vi "UI.vi"(8 "error":errorcluster, 11 "2-axis":refnum<class "Syncronus 2-Axis Stage.lvclass">) -> (0 "error out":errorcluster)   [LabVIEW 2022 SP3, in "JKI UI.lvlib"]
uses:
  JKI UI.lvlib
  Syncronus 2-Axis Stage/Syncronus 2-Axis Stage.lvclass
panel:
  out "XY Position Graph":cluster{"X":dbl, "Y":dbl}[](graph)
  in  "Clear Error":bool
  in  "Set X-Speed":u16
  in  "Set Y-Speed":u16
  in  "Set X-Acceleration":u16
  in  "Set Y-Acceleration":u16
  out "X-Speed":dbl
  out "Y-Speed":dbl
  out "X-Current Speed":dbl
  out "Y-Current Speed":dbl
  out "X-Acceleration":dbl
  out "Y-Acceleration":dbl
  out "Y-Homed":bool
  out "X-Homed":bool
  out "X-Moving":bool
  out "Y-Moving":bool
  out "Y-Position":dbl
  out "X-Position":dbl
  out "Stage Error":errorcluster
  in  "Abort Motion":bool
  in  "Home Stage":bool
  in  "Move Stage":bool
  in  "Y-Destination":dbl
  in  "X-Destination":dbl
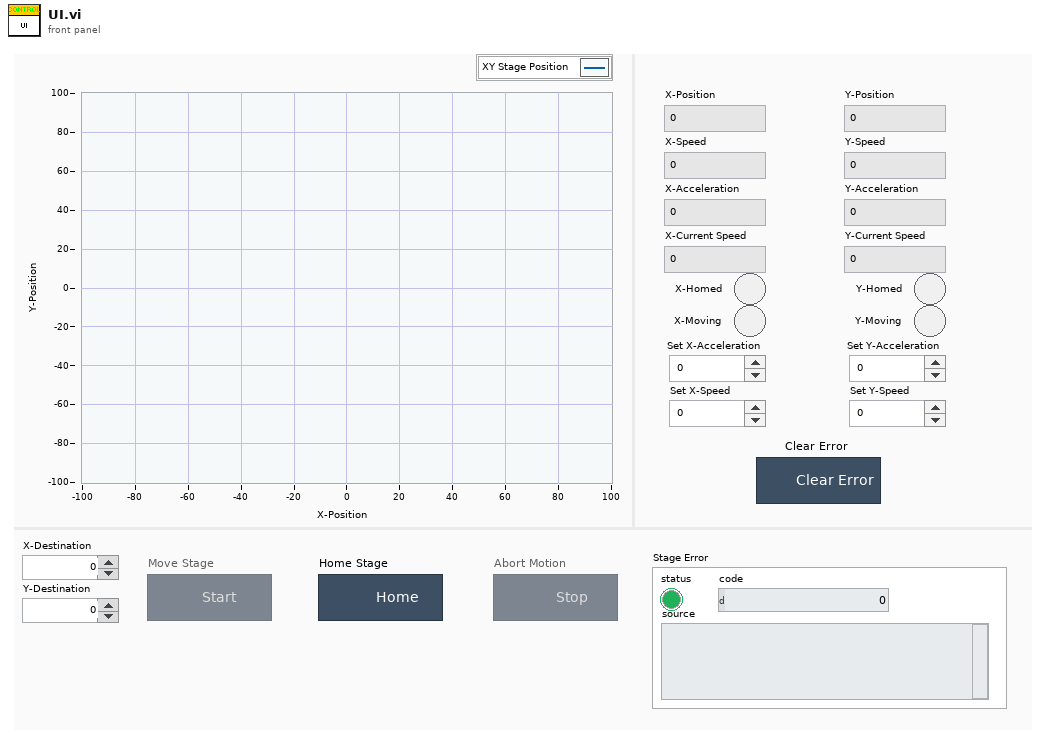
[diagram p1: front panel]
types:
  T1 = enum32{"Invalid", "Standard", "Closed", "Hidden", "Minimized", "Maximized"}
  T2 = enum32{"invalid app kind", "Development System", "Run Time System", "Student Edition", "Embedded LabVIEW", "Evaluation", "Custom"}
  T3 = enum8{"Enabled", "Disabled", "Disabled and Grayed Out"}
  T4 = cluster{"Core":cluster{"Current VI Reference":refnum<vi>, "Close Panel on Exit?":bool}, "2-axis":refnum<class "Syncronus 2-Axis Stage.lvclass">}
  T5 = cluster{"Current VI Reference":refnum<vi>, "Close Panel on Exit?":bool}
  T6 = cluster{"Current Position X":dbl, "Current Position Y":dbl}[]
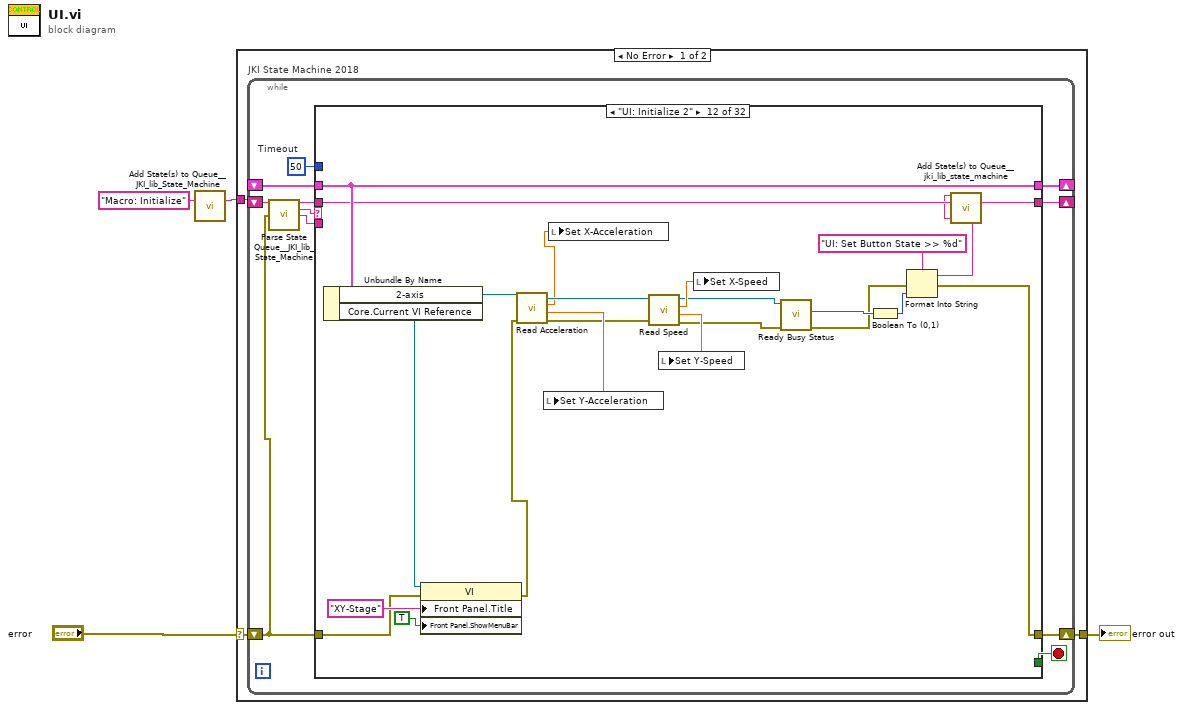
[diagram p0: block diagram]
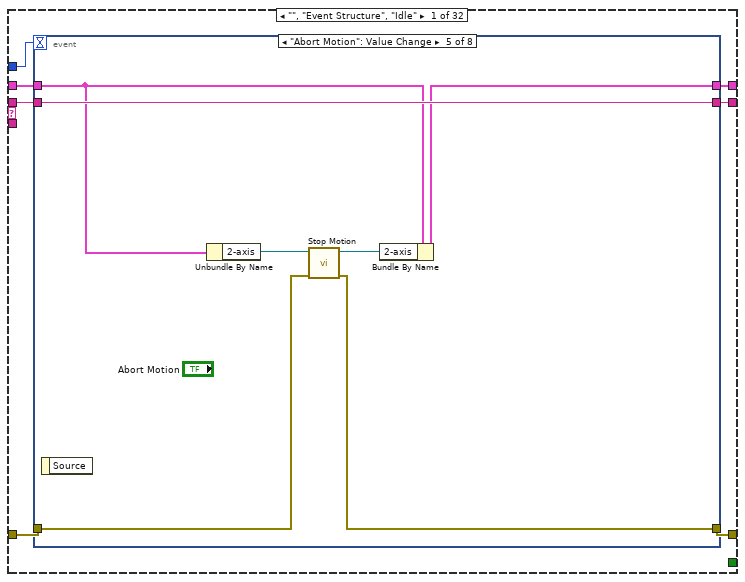
[diagram p2: hidden frame]
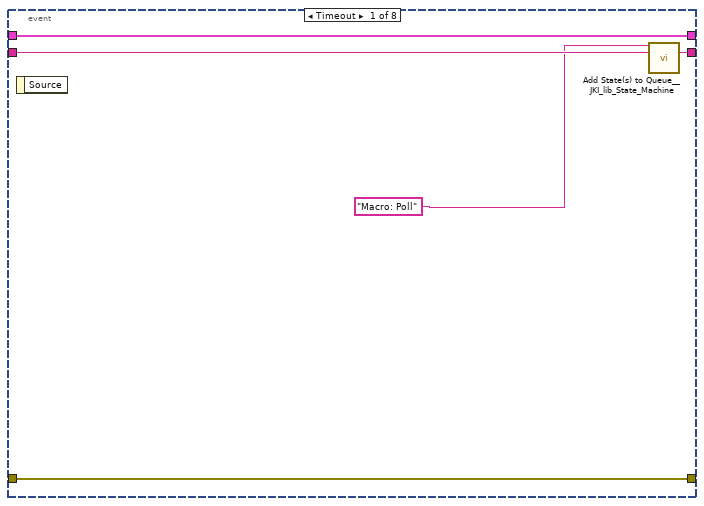
[diagram p3: hidden frame]
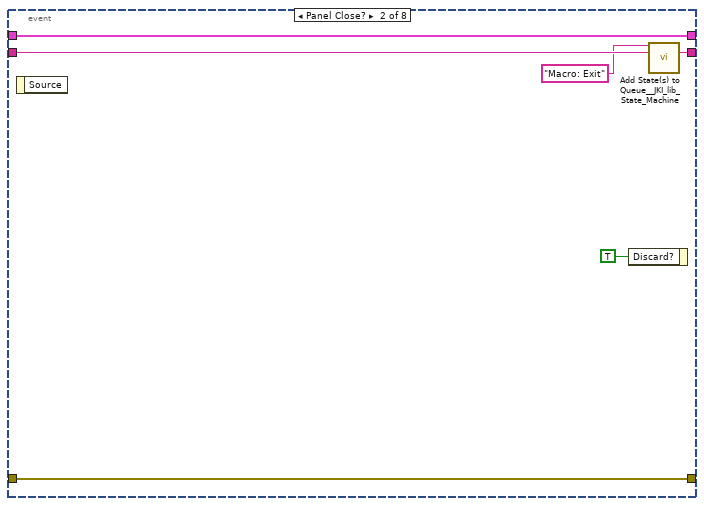
[diagram p4: hidden frame]
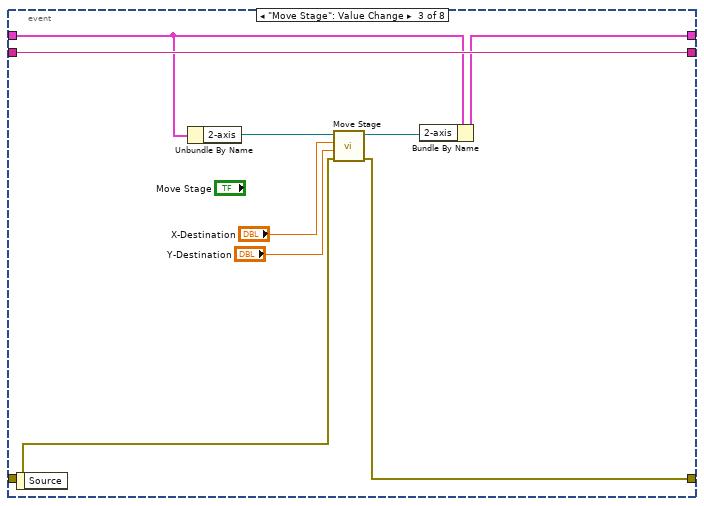
[diagram p5: hidden frame]
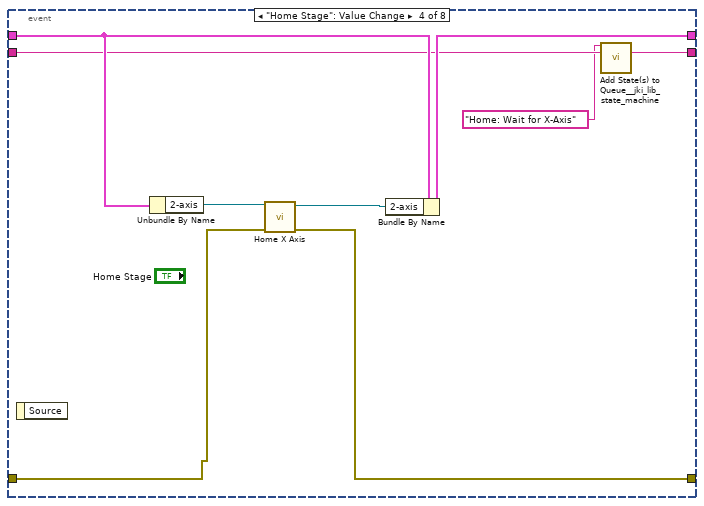
[diagram p6: hidden frame]
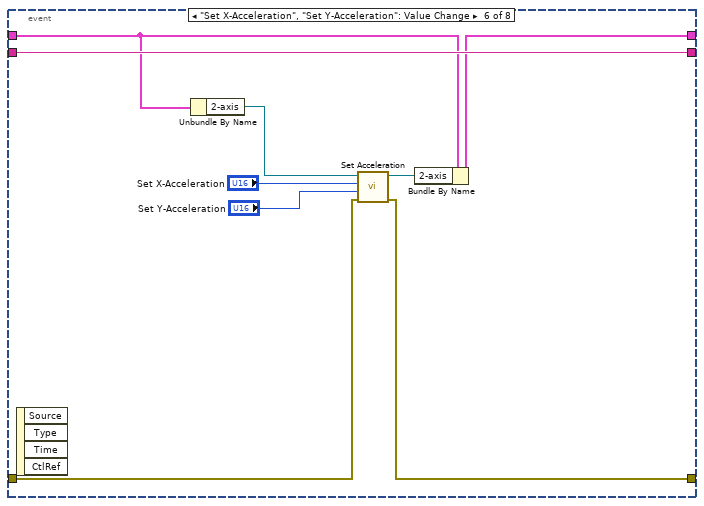
[diagram p7: hidden frame]
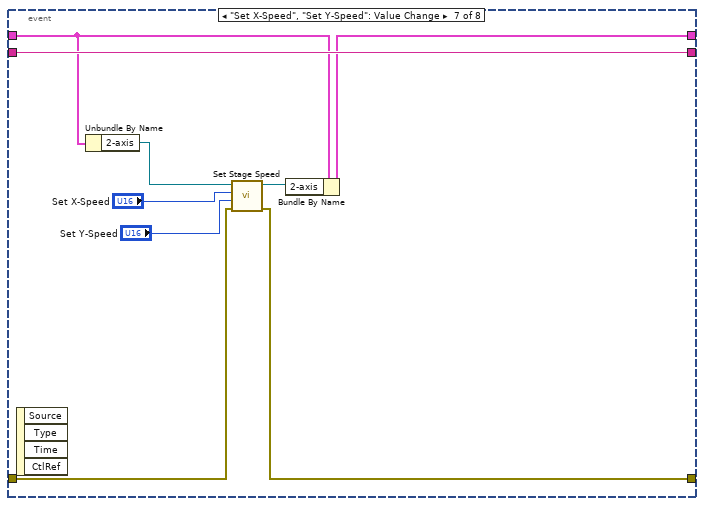
[diagram p8: hidden frame]
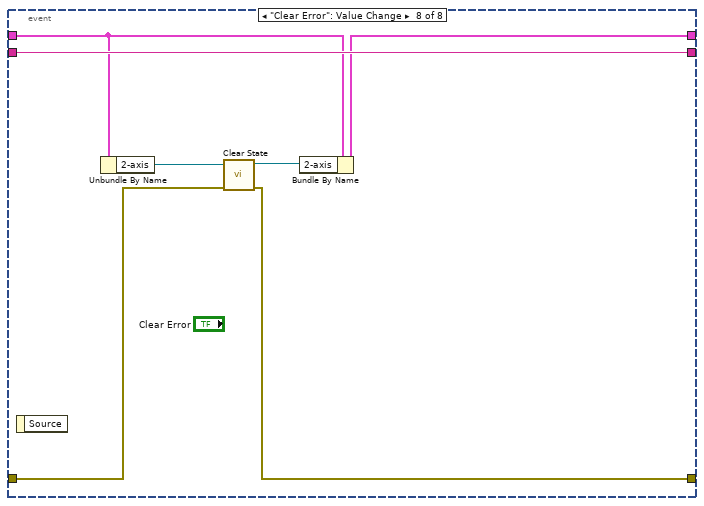
[diagram p9: hidden frame]
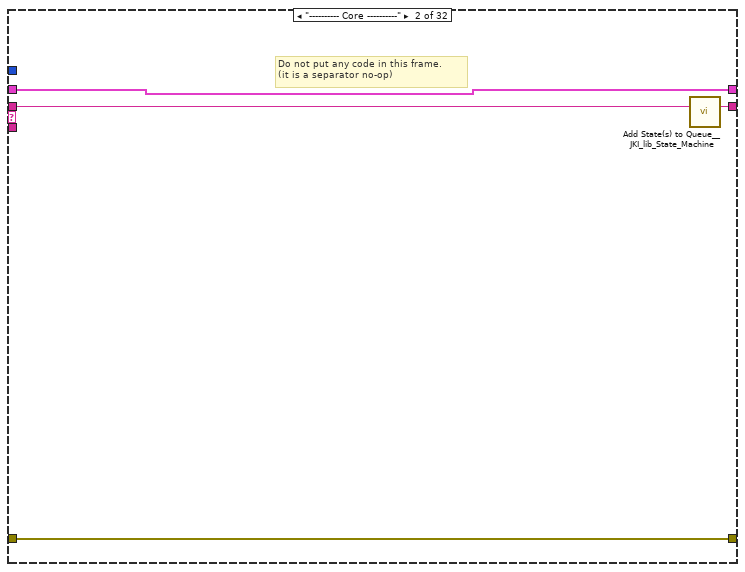
[diagram p10: hidden frame]
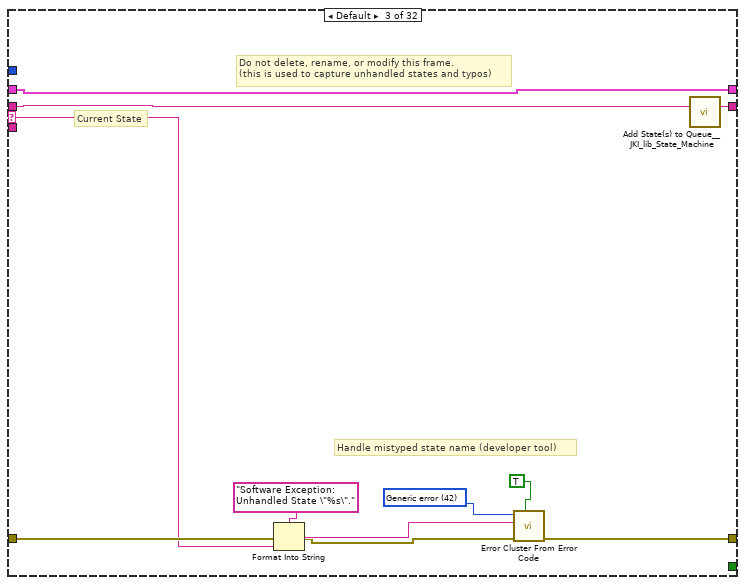
[diagram p11: hidden frame]
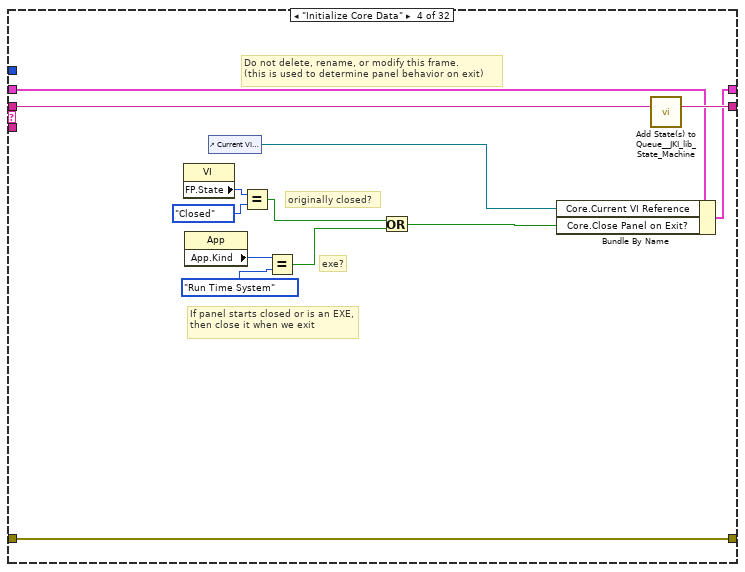
[diagram p12: hidden frame]
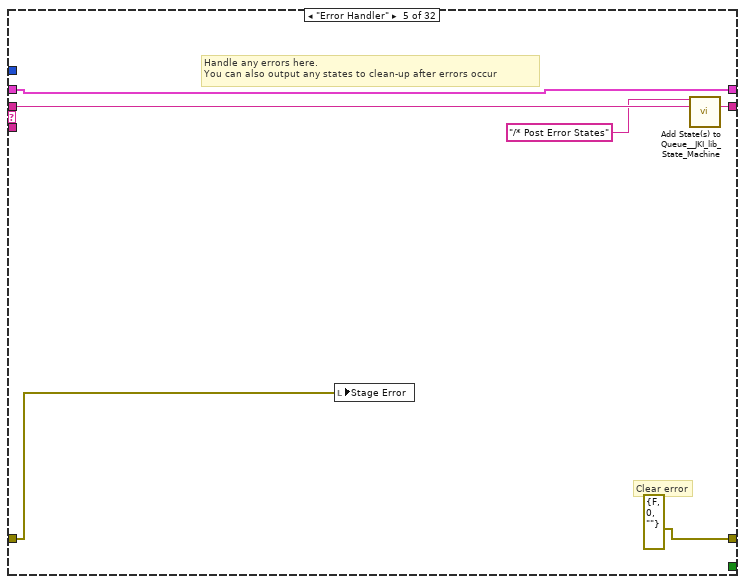
[diagram p13: hidden frame]
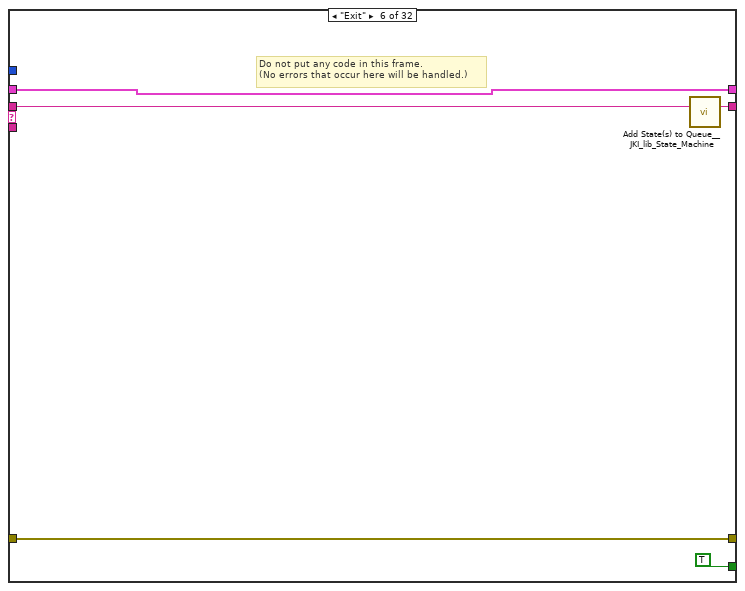
[diagram p14: hidden frame]
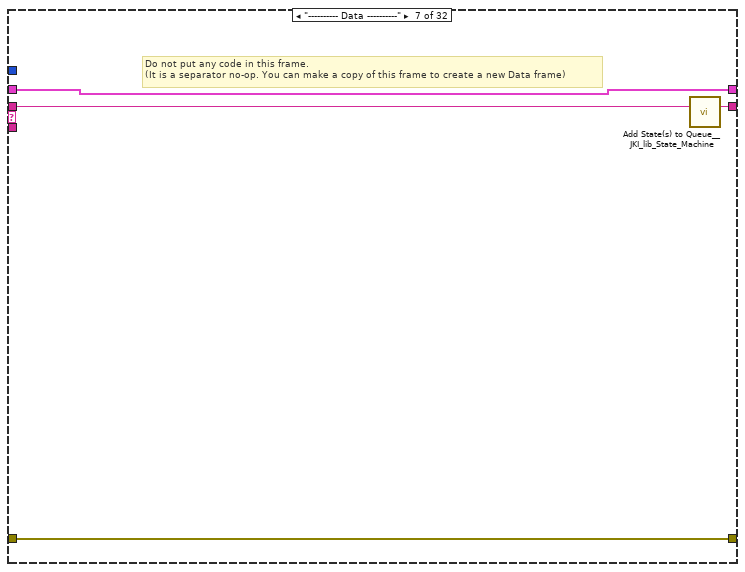
[diagram p15: hidden frame]
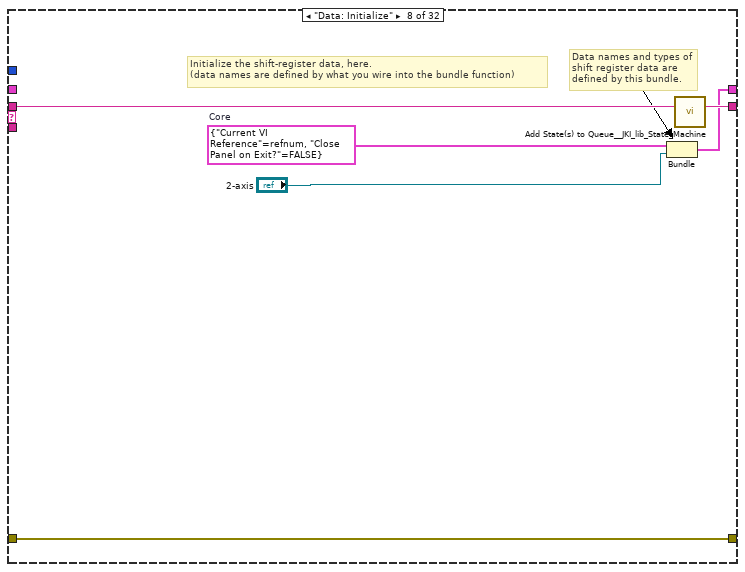
[diagram p16: hidden frame]
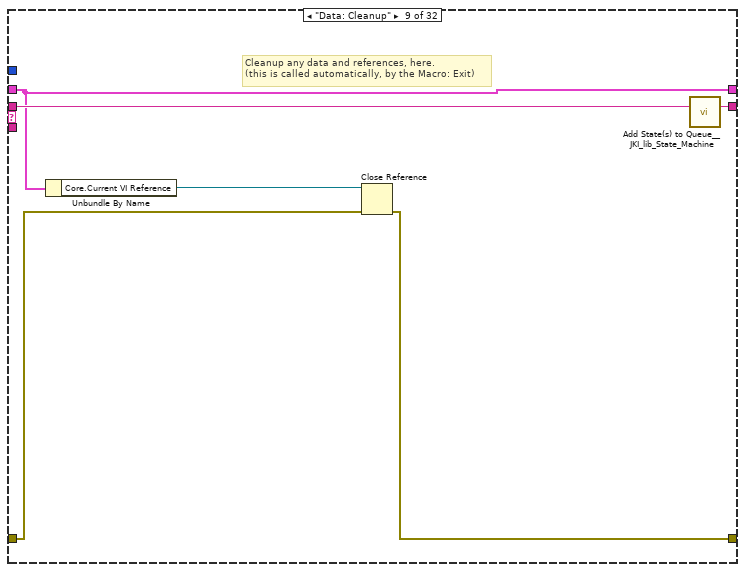
[diagram p17: hidden frame]
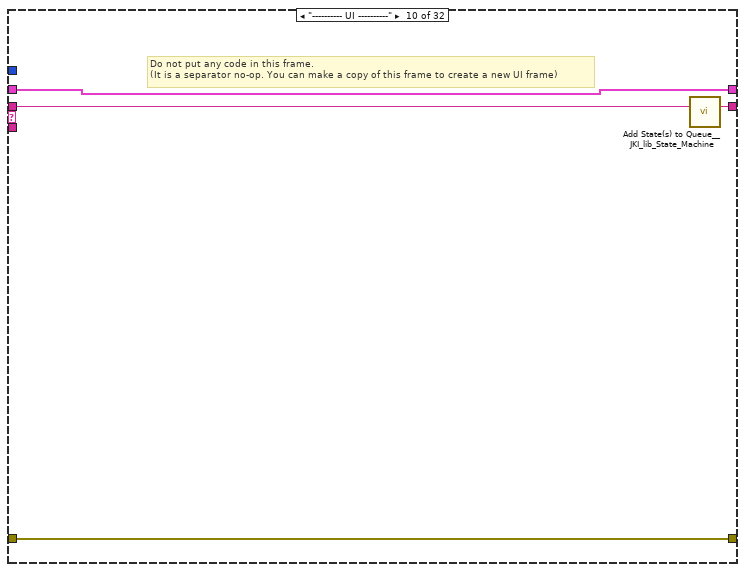
[diagram p18: hidden frame]
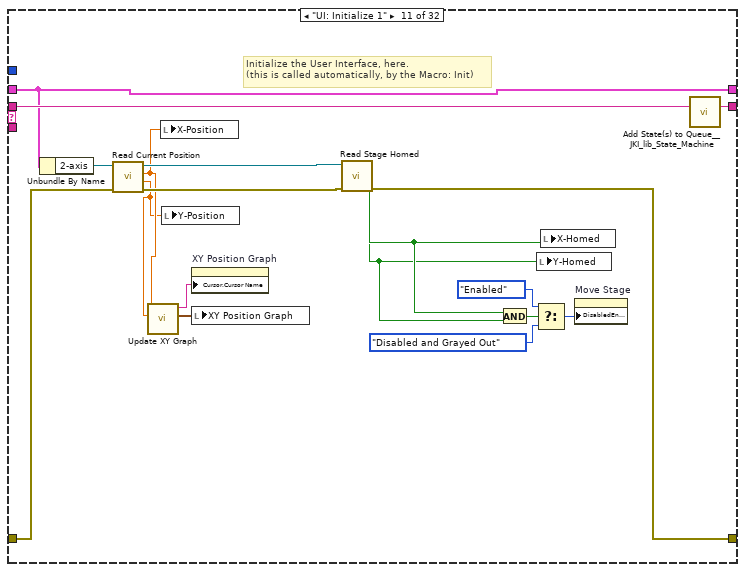
[diagram p19: hidden frame]
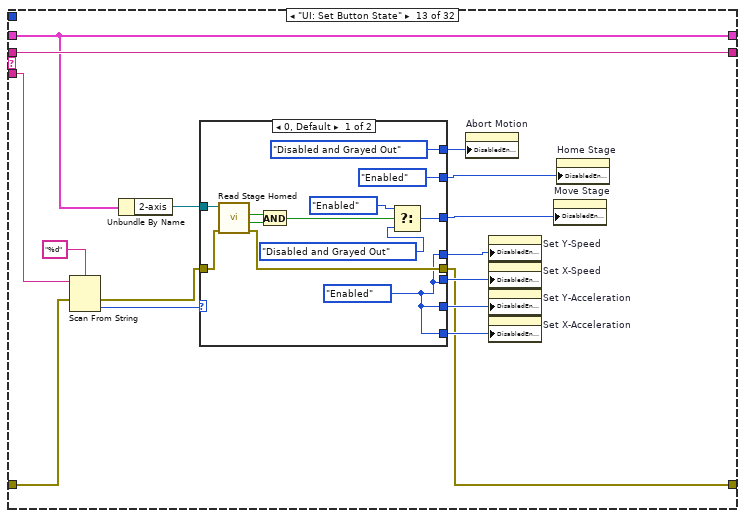
[diagram p20: hidden frame]
diagram:
  n1 = call <vilib>:"Add State(s) to Queue__JKI_lib_State_Machine.vi"("State(s) in (\"\")"="Macro: Initialize") -> ("States Out"=w1:string)  [unwired: 14 in]
  n2 = case shown="No Error" "error" {
    selector: "error" -> [w7 _]
    tunnel: [w6 _] -> w3
    tunnel: w1 -> [w5 _]
    frame No Error {
      n3 = while "JKI State Machine 2018" {
        shift-right: [w11] -> _
        shift-left: _ -> [w10]
        shift-right: [w14] -> w6
        shift-left: w7 -> [w8]
        shift-right: [w13] -> _
        shift-left: w5 -> [w15]
        stop <- w12 stop-if-true
        w9 = 50  # Timeout
        n4 = call <vilib>:"Parse State Queue__JKI_lib_State_Machine.vi"("State Queue"=w15, "Error In (no error)"=w8) -> ("Remaining States"=w17:string, "Current State"=w18:string, "Arguments"=w16:string)  [unwired: 11 in]
        n5 = case shown="\"UI: Initialize 2\"" w18 {
          selector: w18 -> [_ _ w91 _ _ _ _ _ _ _ _ _ _ _ _ _ _ _ _ _ _ _ _ _ _ _ _ _ _ _ _ _]
          tunnel: w17 -> [w25 w90 w95 w114 w120 w125 w129 w135 w141 w145 w163 w184 w202 w223 w234 w303 w308 w318 w321 w326 w338 w347 w356 w365 w374 w380 w395 w403 w406 w413 w433 w442]
          tunnel: w16 -> [_ _ _ _ _ _ _ _ _ _ _ _ w192 w218 w228 _ _ _ _ _ _ _ _ _ _ _ _ _ _ _ _ _]
          tunnel: w10 -> [w23 w87 w93 w107 w117 w123 w126 _ w136 w142 w161 w186 w194 w221 w230 w300 w305 w315 w323 w325 w335 w346 w355 w364 w373 w384 w394 w402 w405 w423 w440 w449]
          tunnel: [w22 w88 w97 w111 errorcluster {"status"=FALSE, "code"=0, "source"=""} ("error out") w122 w127 w132 w137 w143 w151 w165 w189 w219 w231 w301 w306 w316 w319 w324 w329 w341 w350 w359 w368 w377 w391 w398 w404 w409 w425 w446] -> w14
          tunnel: w8 -> [w21 w88 w96 w111 w115 w122 w127 w132 w138 w143 w158 w170 w188 w220 w232 w301 w306 w316 w319 w324 w331 w342 w351 w360 w369 w378 w392 w399 w404 w411 w427 w447]
          tunnel: [w24 w89 w94 w113 w119 w124 w128 w134 w140 w144 w162 w185 w202 w222 w233 w302 w307 w317 w322 w326 w338 w347 w356 w365 w374 w381 w395 w403 w406 w414 w434 w443] -> w13
          tunnel: [_ _ _ _ _ TRUE _ _ _ _ _ _ _ _ _ _ _ _ _ _ _ _ _ _ _ _ _ _ _ _ _ _] -> w12
          tunnel: [w20 w87 w93 w112 w117 w123 w126 w133 w136 w142 w161 w186 w194 w221 w230 w300 w305 w315 w323 w325 w328 w340 w349 w358 w367 w376 w388 w397 w405 w408 w429 w445] -> w11
          tunnel: w9 -> [w19 _ _ _ _ _ _ _ _ _ _ _ _ _ _ _ _ _ _ _ _ _ _ _ _ _ _ _ _ _ _ _]
          frame "", "Event Structure", "Idle" {
            n6 = event shown="[4] \"Abort Motion\": Value Change" {
              selector: _ -> [_ _ _ _ _ _ _ _]
              dyn-events: _ -> [_ _ _ _ _ _ _ _]
              timeout: w19 -> [_ _ _ _ _ _ _ _]
              tunnel: w25 -> [w30 w36 w45 w47 w61 w70 w79 w86]
              tunnel: [w29 w35 w45 w48 w61 w70 w79 w86] -> w24
              tunnel: w23 -> [w27 w33 w44 w54 w60 w69 w78 w85]
              tunnel: [w28 w34 w40 w49 w59 w65 w76 w83] -> w22
              tunnel: w21 -> [w28 w34 w41 w50 w58 w66 w77 w84]
              tunnel: [w27 w33 w38 w53 w56 w63 w72 w81] -> w20
              event Timeout {
                n7 = event-data() -> ()  [unwired: 1 in, 1 out]
                n8 = call <vilib>:"Add State(s) to Queue__JKI_lib_State_Machine.vi"("State(s) in Front (\"\")"="Macro: Poll", "State(s) in (\"\")"=w30) -> ("States Out"=w29:string)  [unwired: 13 in]
              }
              event Panel Close? {
                n9 = event-data() -> ()  [unwired: 1 in, 1 out]
                n10 = event-data("Discard?"=TRUE) -> ()  [unwired: 1 in, 1 out]
                n11 = call <vilib>:"Add State(s) to Queue__JKI_lib_State_Machine.vi"("State(s) in Front (\"\")"="Macro: Exit", "State(s) in (\"\")"=w36) -> ("States Out"=w35:string)  [unwired: 13 in]
              }
              event "Move Stage": Value Change {
                n12 = event-data() -> ()  [unwired: 1 in, 1 out]
                n13 = Unbundle By Name(w44) -> ("2-axis"=w39:refnum<class "Syncronus 2-Axis Stage.lvclass">)
                n14 = call-dynamic "Move Stage.vi"("error in (no error)"=w41, "Y Axis"="Y-Destination", "X Axis"="X-Destination", "2-Axis Stage in"=w39) -> ("error out"=w40:errorcluster, "2-Axis Stage out"=w37:refnum<class "Syncronus 2-Axis Stage.lvclass">)  [unwired: 6 in]
                n15 = Bundle By Name(cluster=w44, "2-axis"=w37) -> (w38:T4)
              }
              event "Home Stage": Value Change {
                n16 = event-data() -> ()  [unwired: 1 in, 1 out]
                n17 = Unbundle By Name(w54) -> ("2-axis"=w52:refnum<class "Syncronus 2-Axis Stage.lvclass">)
                n18 = call-dynamic "Home X Axis.vi"("error in (no error)"=w50, "Synchronous Home in"=w52) -> ("error out"=w49:errorcluster, "Synchronous Home out"=w51:refnum<class "Syncronus 2-Axis Stage.lvclass">)  [unwired: 8 in]
                n19 = Bundle By Name(cluster=w54, "2-axis"=w51) -> (w53:T4)
                n20 = call <vilib>:"Add State(s) to Queue__jki_lib_state_machine.vi"("State(s) in Front (\"\")"="Home: Wait for X-Axis" ("State(s) in Front (\"\")"), "State(s) in (\"\")"=w47) -> ("States Out"=w48:string)  [unwired: 13 in]
              }
              event "Abort Motion": Value Change {
                n21 = event-data() -> ()  [unwired: 1 in, 1 out]
                n22 = Unbundle By Name(w60) -> ("2-axis"=w57:refnum<class "Syncronus 2-Axis Stage.lvclass">)
                n23 = call-dynamic "Stop Motion.vi"("error in (no error)"=w58, "2-Axis Stage in"=w57) -> ("error out"=w59:errorcluster, "2-Axis Stage out"=w55:refnum<class "Syncronus 2-Axis Stage.lvclass">)  [unwired: 8 in]
                n24 = Bundle By Name(cluster=w60, "2-axis"=w55) -> (w56:T4)
              }
              event "Set X-Acceleration", "Set Y-Acceleration": Value Change {
                n25 = event-data() -> ()  [unwired: 1 in, 4 out]
                n26 = Unbundle By Name(w69) -> ("2-axis"=w64:refnum<class "Syncronus 2-Axis Stage.lvclass">)
                n27 = call-dynamic "Set Acceleration.vi"("error in (no error)"=w66, "Y Axis"="Set Y-Acceleration", "X Axis"="Set X-Acceleration", "2-Axis Stage in"=w64) -> ("error out"=w65:errorcluster, "2-Axis Stage out"=w62:refnum<class "Syncronus 2-Axis Stage.lvclass">)  [unwired: 6 in]
                n28 = Bundle By Name(cluster=w69, "2-axis"=w62) -> (w63:T4)
              }
              event "Set X-Speed", "Set Y-Speed": Value Change {
                n29 = event-data() -> ()  [unwired: 1 in, 4 out]
                n30 = Unbundle By Name(w78) -> ("2-axis"=w73:refnum<class "Syncronus 2-Axis Stage.lvclass">)
                n31 = call-dynamic "Set Stage Speed.vi"("error in (no error)"=w77, "Y Axis"="Set Y-Speed", "X Axis"="Set X-Speed", "2-Axis Stage in"=w73) -> ("error out"=w76:errorcluster, "2-Axis Stage out"=w71:refnum<class "Syncronus 2-Axis Stage.lvclass">)  [unwired: 6 in]
                n32 = Bundle By Name(cluster=w78, "2-axis"=w71) -> (w72:T4)
              }
              event "Clear Error": Value Change {
                n33 = event-data() -> ()  [unwired: 1 in, 1 out]
                n34 = Unbundle By Name(w85) -> ("2-axis"=w82:refnum<class "Syncronus 2-Axis Stage.lvclass">)
                n35 = call-dynamic "Clear State.vi"("error in (no error)"=w84, "2-Axis Stage Status in"=w82) -> ("error out"=w83:errorcluster, "2-Axis Stage Status out"=w80:refnum<class "Syncronus 2-Axis Stage.lvclass">)  [unwired: 8 in]
                n36 = Bundle By Name(cluster=w85, "2-axis"=w80) -> (w81:T4)
              }
            }
          }
          frame "---------- Core ----------" {
            # "Do not put any code in this frame.\n(it is a separator no-op)"
            n37 = call <vilib>:"Add State(s) to Queue__JKI_lib_State_Machine.vi"("State(s) in (\"\")"=w90) -> ("States Out"=w89:string)  [unwired: 14 in]
          }
          frame Default {
            w100 = 42 items=["No error", "Argument error", "Memory is full", "Out of zone", "End of file", "File already open", "Generic file I/O error", "File not found", "File permission error", "Disk is full", "Duplicate path", "Too many files open", "System feature not enabled", "Resource file not found", "Cannot add resource", "Resource not found", "Image not found", "Image memory error", "Pen does not exist", "Config type invalid", "Config token not found", "Config parse error", "Config memory error", "Bad external code format", "Bad external code offset", "External code not present", "Null window", "Destroy window error", "Null menu", "Print aborted", "Bad print record", "Print driver error", "Windows error during printing", "Memory error during printing", "Print dialog error", "Generic print error", "Invalid device refnum", "Device not found", "Device parameter error", "Device unit error", "Cannot open device", "Device call aborted", "Generic error", "Cancelled by user", "Object ID too low", "Object ID too high", "Object not in heap", "Unknown heap", "Unknown object (invalid DefProc)", "Unknown object (DefProc not in table)", "Message out of range", "Invalid (null) method", "Unknown message", "Manager call not supported", "Bad address", "Network operation in progress", "Network operation timed out", "Connection is busy", "Network attribute not supported", "Network error", "Address in use", "System out of memory", "Connection aborted", "Connection refused", "Not connected", "Already connected", "Connection closed", "Initialization error (interapplication manager)", "Bad occurrence", "Wait on unbound occurrence handler", "Occurrence queue overflow", "Datalog type conflict", "Unused", "Unrecognized type (interapplication manager)", "Memory corrupt", "Failed to make temporary DLL", "Old CIN version", "Drag socket not found", "Failed to load drop-object", "Failed to register OLE object", "Failed to release OLE object", "Format specifier type mismatch", "Unknown format specifier", "Too few format specifiers", "Too many format specifiers", "Scan failed", "Newer CIN version", "Error converting to variant", "Runtime menu error", "Password tampered", "Variant attribute not found", "Incompatible variant data type", "Event data is not available", "Event Store is not present", "Occurrence is not found", "Event Queue is not created", "Event info is not available", "Refnum passed is NULL", "Error retrieving Class GUID", "Error retrieving CoClass GUID", "Error retrieving TypeLib GUID.", "Bad built application magic bytes.", "Specific driver is different from the specific driver associated with the Logical Name.", "There is no session opened to the class driver.", "Max Error", "MAX - Error with config objects", "MAX - Error loading configuration", "MAX - Group not supported"]
            # "Current State"
            # "Do not delete, rename, or modify this frame.\n(this is used to capture unhandled states and typos)"
            # "Handle mistyped state name (developer tool)"
            n38 = Format Into String(format string="Software Exception: Unhandled State \"%s\"." ("message"), error in=w96, w91) -> (resulting string=w99:string, error out=w98:errorcluster)  [unwired: 1 in]
            n39 = call <vilib>:"Error Cluster From Error Code.vi"("show call chain? (False)"=TRUE, "error in (no error)"=w98, "error message (\"\")"=w99, "error code (0)"=w100) -> ("error out"=w97:errorcluster)  [unwired: 5 in]
            n40 = call <vilib>:"Add State(s) to Queue__JKI_lib_State_Machine.vi"("State(s) in (\"\")"=w95) -> ("States Out"=w94:string)  [unwired: 14 in]
          }
          frame "Initialize Core Data" {
            # "Do not delete, rename, or modify this frame.\n(this is used to determine panel behavior on exit)"
            # "originally closed?"
            # "exe?"
            # "If panel starts closed or is an EXE, then close it when we exit"
            n41 = property class="VI"() -> ("FP.State"=w104:T1)  [unwired: 2 in, 2 out]
            n42 = property class="App"() -> ("App.Kind"=w110:T2)  [unwired: 2 in, 2 out]
            n43 = control-ref of="Current VI Reference"() -> (w105:refnum<vi>)
            n44 = Equal?(x=w104, y=T1."Closed" ("Front Panel Window:State")) -> (x = y?=w102:bool)
            n45 = Equal?(x=w110, y=T2."Run Time System" ("Application:Kind")) -> (x = y?=w108:bool)
            n46 = Or(x=w102, y=w108) -> (x .or. y?=w106:bool)
            n47 = Bundle By Name(cluster=w107, "Core.Current VI Reference"=w105, "Core.Close Panel on Exit?"=w106) -> (w112:T4)
            n48 = call <vilib>:"Add State(s) to Queue__JKI_lib_State_Machine.vi"("State(s) in (\"\")"=w114) -> ("States Out"=w113:string)  [unwired: 14 in]
          }
          frame "Error Handler" {
            # "Handle any errors here.\nYou can also output any states to clean-up after errors occur"
            # "Clear error"
            n49 = local write "Stage Error"(w115) -> ()
            n50 = call <vilib>:"Add State(s) to Queue__JKI_lib_State_Machine.vi"("State(s) in Front (\"\")"="/* Post Error States", "State(s) in (\"\")"=w120) -> ("States Out"=w119:string)  [unwired: 13 in]
          }
          frame "Exit" {
            # "Do not put any code in this frame.\n(No errors that occur here will be handled.)"
            n51 = call <vilib>:"Add State(s) to Queue__JKI_lib_State_Machine.vi"("State(s) in (\"\")"=w125) -> ("States Out"=w124:string)  [unwired: 14 in]
          }
          frame "---------- Data ----------" {
            # "Do not put any code in this frame.\n(It is a separator no-op. You can make a copy of this frame to create a new Data frame)"
            n52 = call <vilib>:"Add State(s) to Queue__JKI_lib_State_Machine.vi"("State(s) in (\"\")"=w129) -> ("States Out"=w128:string)  [unwired: 14 in]
          }
          frame "Data: Initialize" {
            w131 = T5 {"Current VI Reference"=refnum, "Close Panel on Exit?"=FALSE}  # Core
            # "Data names and types of shift register data are defined by this bundle."
            # "Initialize the shift-register data, here.\n(data names are defined by what you wire into the bundle function)"
            n53 = Bundle("Core"=w131, "2-axis"="2-axis") -> (w133:T4)  [unwired: 1 in]
            n54 = call <vilib>:"Add State(s) to Queue__JKI_lib_State_Machine.vi"("State(s) in (\"\")"=w135) -> ("States Out"=w134:string)  [unwired: 14 in]
          }
          frame "Data: Cleanup" {
            # "Cleanup any data and references, here.\n(this is called automatically, by the Macro: Exit)"
            n55 = Unbundle By Name(w136) -> ("Core.Current VI Reference"=w139:refnum<vi>)
            n56 = Close Reference(reference=w139, error in (no error)=w138) -> (error out=w137:errorcluster)
            n57 = call <vilib>:"Add State(s) to Queue__JKI_lib_State_Machine.vi"("State(s) in (\"\")"=w141) -> ("States Out"=w140:string)  [unwired: 14 in]
          }
          frame "---------- UI ----------" {
            # "Do not put any code in this frame.\n(It is a separator no-op. You can make a copy of this frame to create a new UI frame)"
            n58 = call <vilib>:"Add State(s) to Queue__JKI_lib_State_Machine.vi"("State(s) in (\"\")"=w145) -> ("States Out"=w144:string)  [unwired: 14 in]
          }
          frame "UI: Initialize 1" {
            # "Initialize the User Interface, here.\n(this is called automatically, by the Macro: Init)"
            n59 = Unbundle By Name(w161) -> ("2-axis"=w146:refnum<class "Syncronus 2-Axis Stage.lvclass">)
            n60 = call-dynamic "Read Current Position.vi"("error in (no error)"=w158, "2-Axis Stage Status in"=w146) -> ("error out"=w159:errorcluster, "Y Position"=w149:dbl, "X Position"=w150:dbl, "2-Axis Stage Status out"=w160:refnum<class "Syncronus 2-Axis Stage.lvclass">)  [unwired: 6 in]
            n61 = call "Update XY Graph.vi"("Current Position Y"=w149, "Current Position X"=w150) -> ("Array"=w148:T6, "String"=w147:string)  [unwired: 7 in, 1 out]
            n62 = local write "X-Position"(w150) -> ()
            n63 = local write "Y-Position"(w149) -> ()
            n64 = property on="XY Position Graph" class="XYGraph (strict)"("Cursor.Cursor Name"=w147) -> ()  [unwired: 2 in, 2 out]
            n65 = local write "XY Position Graph"(w148) -> ()
            n66 = call-dynamic "Read Stage Homed.vi"("error in (no error)"=w159, "2-Axis Stage Status in"=w160) -> ("error out"=w151:errorcluster, "Y-Axis Homed Moving"=w156:bool, "X-Axis Homed"=w157:bool)  [unwired: 6 in, 1 out]
            n67 = And(x=w157, y=w156) -> (x .and. y?=w155:bool)
            n68 = Select(t=T3."Enabled" ("Disabled"), s=w155, f=T3."Disabled and Grayed Out" ("Disabled")) -> (s? t:f=w153:T3)
            n69 = local write "Y-Homed"(w156) -> ()
            n70 = local write "X-Homed"(w157) -> ()
            n71 = property on="Move Stage" class="Bool"("DisabledEnum"=w153) -> ()  [unwired: 2 in, 2 out]
            n72 = call <vilib>:"Add State(s) to Queue__JKI_lib_State_Machine.vi"("State(s) in (\"\")"=w163) -> ("States Out"=w162:string)  [unwired: 14 in]
          }
          frame "UI: Initialize 2" {
            n73 = Unbundle By Name(w186) -> ("2-axis"=w176:refnum<class "Syncronus 2-Axis Stage.lvclass">, "Core.Current VI Reference"=w179:refnum<vi>)
            n74 = property class="VI"(reference=w179, error in=w170, "Front Panel.Title"="XY-Stage" ("Front Panel Window:Title"), "Front Panel.ShowMenuBar"=TRUE ("Front Panel Window:Show Menu Bar")) -> (error out=w169:errorcluster)  [unwired: 1 out]
            n75 = call-dynamic "Read Acceleration.vi"("error in (no error)"=w169, "2-Axis Stage Status in"=w176) -> ("error out"=w168:errorcluster, "Y Acceleration"=w173:dbl, "X Acceleration"=w174:dbl, "2-Axis Stage Status out"=w175:refnum<class "Syncronus 2-Axis Stage.lvclass">)  [unwired: 6 in]
            n76 = local write "Set Y-Acceleration"(w173) -> ()
            n77 = local write "Set X-Acceleration"(w174) -> ()
            n78 = call-dynamic "Read Speed.vi"("error in (no error)"=w168, "2-Axis Stage Status in"=w175) -> ("error out"=w167:errorcluster, "Y-Axis Speed"=w171:dbl, "X-Axis Speed"=w172:dbl, "2-Axis Stage Status out"=w164:refnum<class "Syncronus 2-Axis Stage.lvclass">)  [unwired: 6 in]
            n79 = local write "Set Y-Speed"(w171) -> ()
            n80 = local write "Set X-Speed"(w172) -> ()
            n81 = call-dynamic "Ready Busy Status.vi"("error in (no error)"=w167, "2-Axis Stage Status in"=w164) -> ("error out"=w166:errorcluster, "Busy"=w181:bool)  [unwired: 7 in, 1 out]
            n82 = Boolean To (0,1)(Boolean=w181) -> (0, 1=w180:i16)
            n83 = Format Into String(format string="UI: Set Button State >> %d", error in=w166, w180) -> (resulting string=w182:string, error out=w165:errorcluster)  [unwired: 1 in]
            n84 = call <vilib>:"Add State(s) to Queue__jki_lib_state_machine.vi"("State(s) in Front (\"\")"=w182, "State(s) in (\"\")"=w184) -> ("States Out"=w185:string)  [unwired: 13 in]
          }
          frame "UI: Set Button State" {
            n85 = Scan From String(format string="%d", input string=w192, error in=w188) -> (error out=w187:errorcluster, output 1=w190:i32)  [unwired: 2 in, 2 out]
            n86 = Unbundle By Name(w194) -> ("2-axis"=w193:refnum<class "Syncronus 2-Axis Stage.lvclass">)
            n87 = case shown="0, Default" w190 {
              tunnel: [T3."Enabled" ("Disabled") w216] -> w201
              tunnel: [T3."Disabled and Grayed Out" ("Disabled") T3."Enabled" ("Disabled")] -> w200
              tunnel: [w207 w216] -> w199
              tunnel: [w206 w215] -> w189
              tunnel: [w205 w216] -> w198
              tunnel: [w205 w216] -> w197
              tunnel: [w205 w216] -> w196
              tunnel: [w205 w216] -> w195
              tunnel: w193 -> [w203 _]
              tunnel: w187 -> [w204 w215]
              frame 0, Default {
                w205 = T3."Enabled" ("Disabled")
                n88 = call-dynamic "Read Stage Homed.vi"("error in (no error)"=w204, "2-Axis Stage Status in"=w203) -> ("error out"=w206:errorcluster, "Y-Axis Homed Moving"=w211:bool, "X-Axis Homed"=w212:bool)  [unwired: 6 in, 1 out]
                n89 = And(x=w212, y=w211) -> (x .and. y?=w210:bool)
                n90 = Select(t=T3."Enabled" ("Disabled"), s=w210, f=T3."Disabled and Grayed Out" ("Disabled")) -> (s? t:f=w207:T3)
              }
              frame 1 {
                w216 = T3."Disabled and Grayed Out" ("Disabled")
              }
            }
            n91 = property on="Abort Motion" class="Bool"("DisabledEnum"=w200) -> ()  [unwired: 2 in, 2 out]
            n92 = property on="Set Y-Speed" class="DigNum (strict)"("DisabledEnum"=w198) -> ()  [unwired: 2 in, 2 out]
            n93 = property on="Set X-Speed" class="DigNum (strict)"("DisabledEnum"=w197) -> ()  [unwired: 2 in, 2 out]
            n94 = property on="Set Y-Acceleration" class="DigNum (strict)"("DisabledEnum"=w196) -> ()  [unwired: 2 in, 2 out]
            n95 = property on="Set X-Acceleration" class="DigNum (strict)"("DisabledEnum"=w195) -> ()  [unwired: 2 in, 2 out]
            n96 = property on="Move Stage" class="Bool"("DisabledEnum"=w199) -> ()  [unwired: 2 in, 2 out]
            n97 = property on="Home Stage" class="Bool"("DisabledEnum"=w201) -> ()  [unwired: 2 in, 2 out]
          }
          frame "UI: Cursor Set" {
            # "Argument"
            # "Set and Unset Cursor Busy.\n(Usage: \"UI: Cursor Set >> Busy|Idle\")"
            n98 = case shown="\"Idle\", Default" w218 {
              tunnel: w220 -> [w225 w227]
              tunnel: [w224 w226] -> w219
              frame "Idle", Default {
                n99 = call <vilib>:"Unset Busy.vi"("error in (no error)"=w225) -> ("error out"=w224:errorcluster)  [unwired: 10 in]
              }
              frame "Busy" {
                n100 = call <vilib>:"Set Busy.vi"("error in (no error)"=w227) -> ("error out"=w226:errorcluster)  [unwired: 9 in, 1 out]
              }
            }
            n101 = call <vilib>:"Add State(s) to Queue__JKI_lib_State_Machine.vi"("State(s) in (\"\")"=w223) -> ("States Out"=w222:string)  [unwired: 14 in]
          }
          frame "UI: Front Panel State" {
            # "Argument"
            # "Set Front Panel Open or Closed\n(Usage: \"UI: Front Panel State >> Open|Close\")"
            n102 = Unbundle By Name(w230) -> ("Core.Current VI Reference"=w229:refnum<vi>)
            n103 = case shown="\"Minimize\", \"Minimized\"" w228 {
              tunnel: w232 -> [w240 w255 w266 w279 w292]
              tunnel: [w242 w256 w268 w281 w294] -> w231
              tunnel: w229 -> [w241 w253 w267 w280 w293]
              frame "Open", "Standard", Default {
                w235 = T1."Standard" ("State")
                n104 = property class="VI"(reference=w241, error in=w240) -> (reference out=w238:refnum<vi>, error out=w239:errorcluster, "FP.State"=w237:T1)
                n105 = Not Equal?(x=w237, y=w235) -> (x != y?=w236:bool)
                n106 = case shown="True" w236 {
                  tunnel: [w246 w248] -> w242
                  tunnel: w239 -> [w245 w248]
                  tunnel: w238 -> [w244 _]
                  tunnel: w235 -> [w243 _]
                  frame True {
                    n107 = invoke class="VI" method="FP.Open"(reference=w244, error in=w245, "Activate"=TRUE, "State"=w243) -> (error out=w246:errorcluster)  [unwired: 1 in, 4 out]
                  }
                  frame False {
                  }
                }
              }
              frame "Close", "Closed" {
                n108 = property class="VI"(reference=w253, error in=w255) -> (reference out=w252:refnum<vi>, error out=w254:errorcluster, "FP.State"=w250:T1)
                n109 = Not Equal?(x=w250, y=T1."Closed" ("Front Panel Window:State")) -> (x != y?=w249:bool)
                n110 = case shown="True" w249 {
                  tunnel: [w257 w260] -> w256
                  tunnel: w254 -> [w257 w259]
                  tunnel: w252 -> [_ w258]
                  frame False {
                  }
                  frame True {
                    n111 = invoke class="VI" method="FP.Close"(reference=w258, error in=w259) -> (error out=w260:errorcluster)  [unwired: 1 in, 2 out]
                  }
                }
              }
              frame "Hidden", "Hide" {
                w261 = T1."Hidden" ("State")
                n112 = property class="VI"(reference=w267, error in=w266) -> (reference out=w264:refnum<vi>, error out=w265:errorcluster, "FP.State"=w263:T1)
                n113 = Not Equal?(x=w263, y=w261) -> (x != y?=w262:bool)
                n114 = case shown="True" w262 {
                  tunnel: [w272 w273] -> w268
                  tunnel: w265 -> [w271 w273]
                  tunnel: w264 -> [w270 _]
                  tunnel: w261 -> [w269 _]
                  frame True {
                    n115 = invoke class="VI" method="FP.Open"(reference=w270, error in=w271, "State"=w269) -> (error out=w272:errorcluster)  [unwired: 2 in, 4 out]
                  }
                  frame False {
                  }
                }
              }
              frame "Minimize", "Minimized" {
                w274 = T1."Minimized" ("State")
                n116 = property class="VI"(reference=w280, error in=w279) -> (reference out=w277:refnum<vi>, error out=w278:errorcluster, "FP.State"=w276:T1)
                n117 = Not Equal?(x=w276, y=w274) -> (x != y?=w275:bool)
                n118 = case shown="True" w275 {
                  tunnel: [w285 w286] -> w281
                  tunnel: w278 -> [w284 w286]
                  tunnel: w277 -> [w283 _]
                  tunnel: w274 -> [w282 _]
                  frame True {
                    n119 = invoke class="VI" method="FP.Open"(reference=w283, error in=w284, "State"=w282) -> (error out=w285:errorcluster)  [unwired: 2 in, 4 out]
                  }
                  frame False {
                  }
                }
              }
              frame "Maximize", "Maximized" {
                w287 = T1."Maximized" ("State")
                n120 = property class="VI"(reference=w293, error in=w292) -> (reference out=w290:refnum<vi>, error out=w291:errorcluster, "FP.State"=w289:T1)
                n121 = Not Equal?(x=w289, y=w287) -> (x != y?=w288:bool)
                n122 = case shown="True" w288 {
                  tunnel: [w298 w299] -> w294
                  tunnel: w291 -> [w297 w299]
                  tunnel: w290 -> [w296 _]
                  tunnel: w287 -> [w295 _]
                  frame True {
                    n123 = invoke class="VI" method="FP.Open"(reference=w296, error in=w297, "State"=w295) -> (error out=w298:errorcluster)  [unwired: 2 in, 4 out]
                  }
                  frame False {
                  }
                }
              }
            }
            n124 = call <vilib>:"Add State(s) to Queue__JKI_lib_State_Machine.vi"("State(s) in (\"\")"=w234) -> ("States Out"=w233:string)  [unwired: 14 in]
          }
          frame "---------- Macro ----------" {
            # "Do not put any code in this frame.\n(It is a separator no-op. You can make a copy of this frame to create a new Macro frame)"
            n125 = call <vilib>:"Add State(s) to Queue__JKI_lib_State_Machine.vi"("State(s) in (\"\")"=w303) -> ("States Out"=w302:string)  [unwired: 14 in]
          }
          frame "Macro: Initialize" {
            w304 = "Data: Initialize\nInitialize Core Data\nUI: Initialize 1\nUI: Initialize 2\nUI: Front Panel State >> Open"  # Data: Initialize Initialize Core Data UI: Initialize 1 UI: Initialize 2 UI: Front Panel State >> Open
            # "Initialization Macro\n(This is called once, when the VI starts)"
            n126 = call <vilib>:"Add State(s) to Queue__JKI_lib_State_Machine.vi"("State(s) in Front (\"\")"=w304, "State(s) in (\"\")"=w308) -> ("States Out"=w307:string)  [unwired: 13 in]
          }
          frame "Macro: Exit" {
            # "Exit Macro\n(This is called once, when the VI exits)"
            n127 = Unbundle By Name(w315) -> ("Core.Close Panel on Exit?"=w314:bool)
            n128 = Select(t="UI: Front Panel State >> Close", s=w314, f="") -> (s? t:f=w311:string)
            n129 = call <vilib>:"Add State(s) to Queue__JKI_lib_State_Machine.vi"("State(s) in (\"\")"=w311, "State(s) at Back (\"\")"="Data: Cleanup\nExit") -> ("States Out"=w309:string)  [unwired: 13 in]
            n130 = call <vilib>:"Add State(s) to Queue__JKI_lib_State_Machine.vi"("State(s) in Front (\"\")"=w309, "State(s) in (\"\")"=w318) -> ("States Out"=w317:string)  [unwired: 13 in]
          }
          frame "Macro: Poll" {
            n131 = call <vilib>:"Add State(s) to Queue__jki_lib_state_machine.vi"("State(s) in Front (\"\")"="Stage: Get Latest Position\nStage: Get Moving Status\nStage: Get Homed Status\nStage: Get Acceleration\nStage: Get Current Speed\nStage: Get Busy Status\nStage: Get Speed\nStage: Get Error", "State(s) in (\"\")"=w321) -> ("States Out"=w322:string)  [unwired: 13 in]
          }
          frame "------Stage------" {
          }
          frame "Stage: Get Latest Position" {
            n132 = Unbundle By Name(w335) -> ("2-axis"=w334:refnum<class "Syncronus 2-Axis Stage.lvclass">)
            n133 = call-dynamic "Read Current Position.vi"("error in (no error)"=w331, "2-Axis Stage Status in"=w334) -> ("error out"=w330:errorcluster, "Y Position"=w332:dbl, "X Position"=w333:dbl, "2-Axis Stage Status out"=w327:refnum<class "Syncronus 2-Axis Stage.lvclass">)  [unwired: 6 in]
            "Y-Position" <- w332
            "X-Position" <- w333
            n134 = call "Update XY Graph.vi"("error in (no error)"=w330, "Current Position Y"=w332, "Current Position X"=w333) -> ("error out"=w329:errorcluster, "Array"=→"XY Position Graph":T6, "String"=w336:string)  [unwired: 6 in]
            n135 = property on="XY Position Graph" class="XYGraph (strict)"("Cursor.Cursor Name"=w336) -> ()  [unwired: 2 in, 2 out]
            n136 = Bundle By Name(cluster=w335, "2-axis"=w327) -> (w328:T4)
          }
          frame "Stage: Get Moving Status" {
            n137 = Unbundle By Name(w346) -> ("2-axis"=w345:refnum<class "Syncronus 2-Axis Stage.lvclass">)
            n138 = call-dynamic "Read Moving Flags.vi"("error in (no error)"=w342, "2-Axis Stage Status in"=w345) -> ("error out"=w341:errorcluster, "Y-Axis Moving"=→"Y-Moving":bool, "X-Axis Moving"=→"X-Moving":bool, "2-Axis Stage Status out"=w339:refnum<class "Syncronus 2-Axis Stage.lvclass">)  [unwired: 6 in]
            n139 = Bundle By Name(cluster=w346, "2-axis"=w339) -> (w340:T4)
          }
          frame "Stage: Get Homed Status" {
            n140 = Unbundle By Name(w355) -> ("2-axis"=w354:refnum<class "Syncronus 2-Axis Stage.lvclass">)
            n141 = call-dynamic "Read Stage Homed.vi"("error in (no error)"=w351, "2-Axis Stage Status in"=w354) -> ("error out"=w350:errorcluster, "Y-Axis Homed Moving"=→"Y-Homed":bool, "X-Axis Homed"=→"X-Homed":bool, "2-Axis Stage Status out"=w348:refnum<class "Syncronus 2-Axis Stage.lvclass">)  [unwired: 6 in]
            n142 = Bundle By Name(cluster=w355, "2-axis"=w348) -> (w349:T4)
          }
          frame "Stage: Get Acceleration" {
            n143 = Unbundle By Name(w364) -> ("2-axis"=w363:refnum<class "Syncronus 2-Axis Stage.lvclass">)
            n144 = call-dynamic "Read Acceleration.vi"("error in (no error)"=w360, "2-Axis Stage Status in"=w363) -> ("error out"=w359:errorcluster, "Y Acceleration"=→"Y-Acceleration":dbl, "X Acceleration"=→"X-Acceleration":dbl, "2-Axis Stage Status out"=w357:refnum<class "Syncronus 2-Axis Stage.lvclass">)  [unwired: 6 in]
            n145 = Bundle By Name(cluster=w364, "2-axis"=w357) -> (w358:T4)
          }
          frame "Stage: Get Current Speed" {
            n146 = Unbundle By Name(w373) -> ("2-axis"=w372:refnum<class "Syncronus 2-Axis Stage.lvclass">)
            n147 = call-dynamic "Read Current Speed.vi"("error in (no error)"=w369, "2-Axis Stage Status in"=w372) -> ("error out"=w368:errorcluster, "Y Current Speed"=→"Y-Current Speed":dbl, "X Current Speed"=→"X-Current Speed":dbl, "2-Axis Stage Status out"=w366:refnum<class "Syncronus 2-Axis Stage.lvclass">)  [unwired: 6 in]
            n148 = Bundle By Name(cluster=w373, "2-axis"=w366) -> (w367:T4)
          }
          frame "Stage: Get Busy Status" {
            n149 = Unbundle By Name(w384) -> ("2-axis"=w383:refnum<class "Syncronus 2-Axis Stage.lvclass">)
            n150 = call-dynamic "Ready Busy Status.vi"("error in (no error)"=w378, "2-Axis Stage Status in"=w383) -> ("error out"=w377:errorcluster, "Busy"=w382:bool, "2-Axis Stage Status out"=w375:refnum<class "Syncronus 2-Axis Stage.lvclass">)  [unwired: 7 in]
            n151 = Bundle By Name(cluster=w384, "2-axis"=w375) -> (w376:T4)
            n152 = Select(t="UI: Set Button State >>1", s=w382, f="UI: Set Button State >>0") -> (s? t:f=w379:string)
            n153 = call <vilib>:"Add State(s) to Queue__jki_lib_state_machine.vi"("State(s) in Front (\"\")"=w379, "State(s) in (\"\")"=w380) -> ("States Out"=w381:string)  [unwired: 13 in]
          }
          frame "Stage: Get Speed" {
            n154 = Unbundle By Name(w394) -> ("2-axis"=w393:refnum<class "Syncronus 2-Axis Stage.lvclass">)
            n155 = call-dynamic "Read Speed.vi"("error in (no error)"=w392, "2-Axis Stage Status in"=w393) -> ("error out"=w391:errorcluster, "Y-Axis Speed"=→"Y-Speed":dbl, "X-Axis Speed"=→"X-Speed":dbl, "2-Axis Stage Status out"=w387:refnum<class "Syncronus 2-Axis Stage.lvclass">)  [unwired: 6 in]
            n156 = Bundle By Name(cluster=w394, "2-axis"=w387) -> (w388:T4)
          }
          frame "Stage: Get Error" {
            n157 = Unbundle By Name(w402) -> ("2-axis"=w401:refnum<class "Syncronus 2-Axis Stage.lvclass">)
            n158 = call-dynamic "Read Error.vi"("error in (no error)"=w399, "2-Axis Stage Status in"=w401) -> ("error out"=w398:errorcluster, "Stage Error"=→"Stage Error":errorcluster, "2-Axis Stage Status out"=w396:refnum<class "Syncronus 2-Axis Stage.lvclass">)  [unwired: 7 in]
            n159 = Bundle By Name(cluster=w402, "2-axis"=w396) -> (w397:T4)
          }
          frame "------Home------" {
          }
          frame "Home: Wait for X-Axis" {
            n160 = Unbundle By Name(w423) -> ("2-axis"=w422:refnum<class "Syncronus 2-Axis Stage.lvclass">)
            n161 = call-dynamic "Read Stage Homed.vi"("error in (no error)"=w411, "2-Axis Stage Status in"=w422) -> ("error out"=w410:errorcluster, "X-Axis Homed"=w420:bool, "2-Axis Stage Status out"=w421:refnum<class "Syncronus 2-Axis Stage.lvclass">)  [unwired: 6 in, 1 out]
            n162 = call-dynamic "Read Moving Flags.vi"("error in (no error)"=w410, "2-Axis Stage Status in"=w421) -> ("error out"=w409:errorcluster, "X-Axis Moving"=w419:bool, "2-Axis Stage Status out"=w407:refnum<class "Syncronus 2-Axis Stage.lvclass">)  [unwired: 6 in, 1 out]
            n163 = Not(x=w419) -> (.not. x?=w418:bool)
            n164 = Bundle By Name(cluster=w423, "2-axis"=w407) -> (w408:T4)
            n165 = And(x=w420, y=w418) -> (x .and. y?=w417:bool)
            n166 = Select(t="Home: Home Y-Axis", s=w417, f="idle\nHome: Wait for X-Axis" ("State(s) in Front (\"\")")) -> (s? t:f=w412:string)
            n167 = call <vilib>:"Add State(s) to Queue__jki_lib_state_machine.vi"("State(s) in Front (\"\")"=w412, "State(s) in (\"\")"=w413) -> ("States Out"=w414:string)  [unwired: 13 in]
          }
          frame "Home: Wait for Y-Axis" {
            n168 = Unbundle By Name(w440) -> ("2-axis"=w439:refnum<class "Syncronus 2-Axis Stage.lvclass">)
            n169 = call-dynamic "Read Stage Homed.vi"("error in (no error)"=w427, "2-Axis Stage Status in"=w439) -> ("error out"=w426:errorcluster, "Y-Axis Homed Moving"=w431:bool, "2-Axis Stage Status out"=w438:refnum<class "Syncronus 2-Axis Stage.lvclass">)  [unwired: 6 in, 1 out]
            n170 = call-dynamic "Read Moving Flags.vi"("error in (no error)"=w426, "2-Axis Stage Status in"=w438) -> ("error out"=w425:errorcluster, "Y-Axis Moving"=w430:bool, "2-Axis Stage Status out"=w428:refnum<class "Syncronus 2-Axis Stage.lvclass">)  [unwired: 6 in, 1 out]
            n171 = Not(x=w430) -> (.not. x?=w437:bool)
            n172 = Bundle By Name(cluster=w440, "2-axis"=w428) -> (w429:T4)
            n173 = And(x=w431, y=w437) -> (x .and. y?=w436:bool)
            n174 = Select(t="idle", s=w436, f="idle\nHome: Wait for Y-Axis") -> (s? t:f=w432:string)
            n175 = call <vilib>:"Add State(s) to Queue__jki_lib_state_machine.vi"("State(s) in Front (\"\")"=w432, "State(s) in (\"\")"=w433) -> ("States Out"=w434:string)  [unwired: 13 in]
          }
          frame "Home: Home Y-Axis" {
            n176 = Unbundle By Name(w449) -> ("2-axis"=w448:refnum<class "Syncronus 2-Axis Stage.lvclass">)
            n177 = call-dynamic "Home Y Axis.vi"("error in (no error)"=w447, "Synchronous Home in"=w448) -> ("error out"=w446:errorcluster, "Synchronous Home out"=w444:refnum<class "Syncronus 2-Axis Stage.lvclass">)  [unwired: 8 in]
            n178 = Bundle By Name(cluster=w449, "2-axis"=w444) -> (w445:T4)
            n179 = call <vilib>:"Add State(s) to Queue__jki_lib_state_machine.vi"("State(s) in Front (\"\")"="Home: Wait for Y-Axis" ("State(s) in Front (\"\")"), "State(s) in (\"\")"=w442) -> ("States Out"=w443:string)  [unwired: 13 in]
          }
        }
      }
    }
    frame Error {
    }
  }
  "error out" <- w3
